vi "Chronos TDMS Generate Array Property Names.vi"(8 "error in (no error)":errorcluster, 9 "Element Name":string, 10 "Label":string, 11 "Array Dimensions":i32[](array[numeric])) -> (0 "error out":errorcluster, 2 "Indecies":i32[][](array[numeric]), 3 "Array Property Names":string[](array[string]))   [LabVIEW 2021]
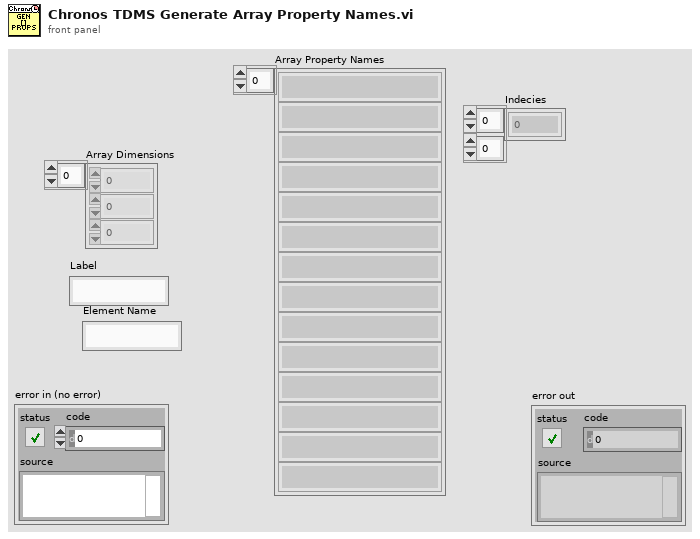
[diagram p1: front panel]
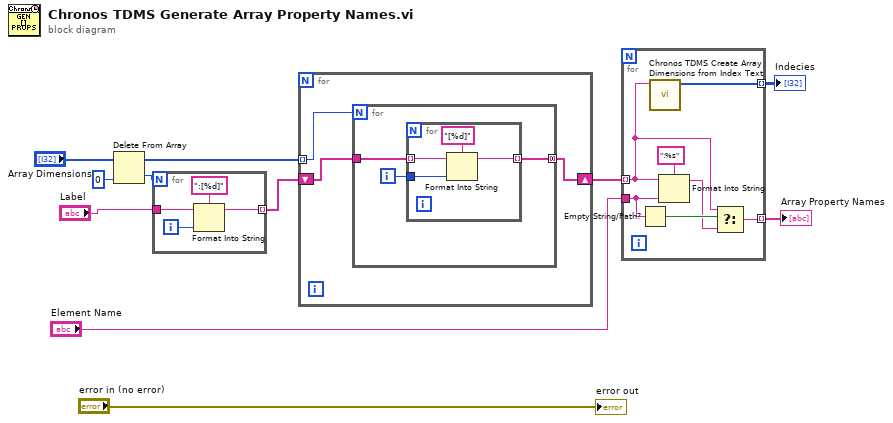
[diagram p0: block diagram]
diagram:
  n1 = Delete From Array(array="Array Dimensions", index=0) -> (deleted portion=w8:i32, array with subset deleted=w10:i32[])  [unwired: 1 in]
  n2 = for {
    N: w8 -> [_]
    tunnel: [w13] -> w7 mode=indexing
    tunnel: "Label" -> [w12]
    i -> [w14]
    n3 = Format Into String(format string=":[%d]", initial string=w12, w14) -> (resulting string=w13:string)  [unwired: 1 in, 1 out]
  }
  n4 = for {
    tunnel: w10 -> [w18] mode=indexing
    shift-right: [w16] -> w5
    shift-left: w7 -> [w17]
    n5 = for {
      N: w18 -> [_]
      tunnel: w17 -> [w21]
      tunnel: [w19] -> w16 mode=concatenating
      i -> [w20]
      n6 = for {
        tunnel: w21 -> [w24] mode=indexing
        tunnel: w20 -> [w23]
        tunnel: [w22] -> w19 mode=indexing
        n7 = Format Into String(format string="[%d]", initial string=w24, w23) -> (resulting string=w22:string)  [unwired: 1 in, 1 out]
      }
    }
  }
  n8 = for {
    tunnel: w5 -> [w26] mode=indexing
    tunnel: "Element Name" -> [w30]
    tunnel: [w27] -> w3 mode=indexing
    tunnel: [w31] -> w1 mode=indexing
    n9 = Empty String/Path?(string/path=w30) -> (empty?=w29:bool)
    n10 = call "Chronos TDMS Create Array Dimensions from Index Text.vi"("index string"=w26) -> ("Indecies"=w31:i32[])  [unwired: 9 in, 1 out]
    n11 = Format Into String(format string=":%s", initial string=w26, w30) -> (resulting string=w28:string)  [unwired: 1 in, 1 out]
    n12 = Select(t=w26, s=w29, f=w28) -> (s? t:f=w27:string)
  }
  "Array Property Names" <- w3
  "Indecies" <- w1
  "error out" <- "error in (no error)"
